vi "ABB configure system.vi"() -> ()   [LabVIEW 2017]
uses:
  ABB global.vi
panel:
  in  "Altitude (m)":dbl
  in  "Max Winding temp Rise (°C)":dbl
  in  "Simulate cDAQ":bool
  in  "Power Analyser":bool
  in  "Exit":bool
  in  "Change password":bool
  in  "Select data Folder":bool
  out "Data Folder":path
  in  "Simulate Norma":bool
  in  "GPIB Addresses":cluster{"Norma 5000":u8, "????":u8}={"Norma 5000"=1, "????"=1} {"????" min=1 max=31; "Norma 5000" min=1 max=31}
  # "Configure System"
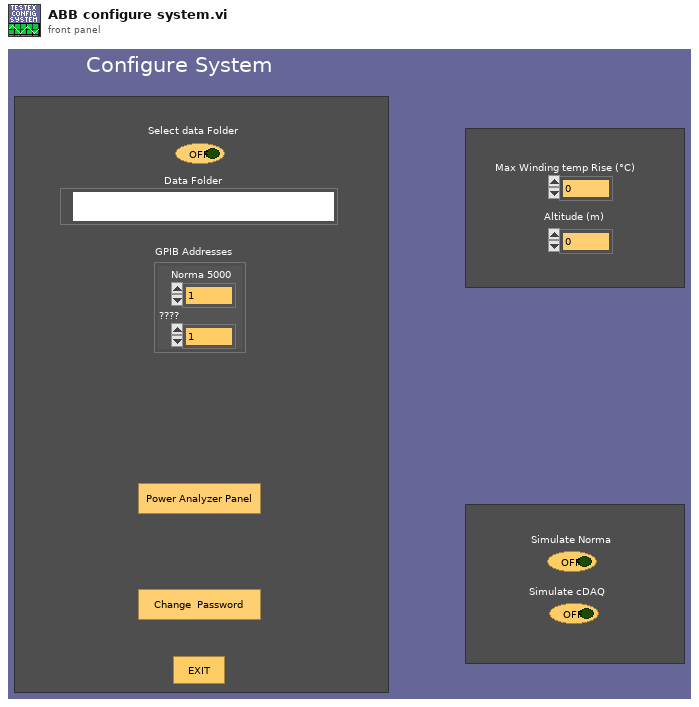
[diagram p1: front panel]
types:
  T1 = cluster{"Simulate Norma":bool, "Norma 5000 Address":u8, "WebDaq IP Address":string, "Simulate cDAQ":bool}
  T2 = enum32{"existing file", "new file", "new or existing file", "existing dir", "new dir", "new or existing dir", "existing file (use LLBs)", "new file (use LLBs)", "new or existing file (use LLBs)", "new or existing file or directory (use LLBs)"}
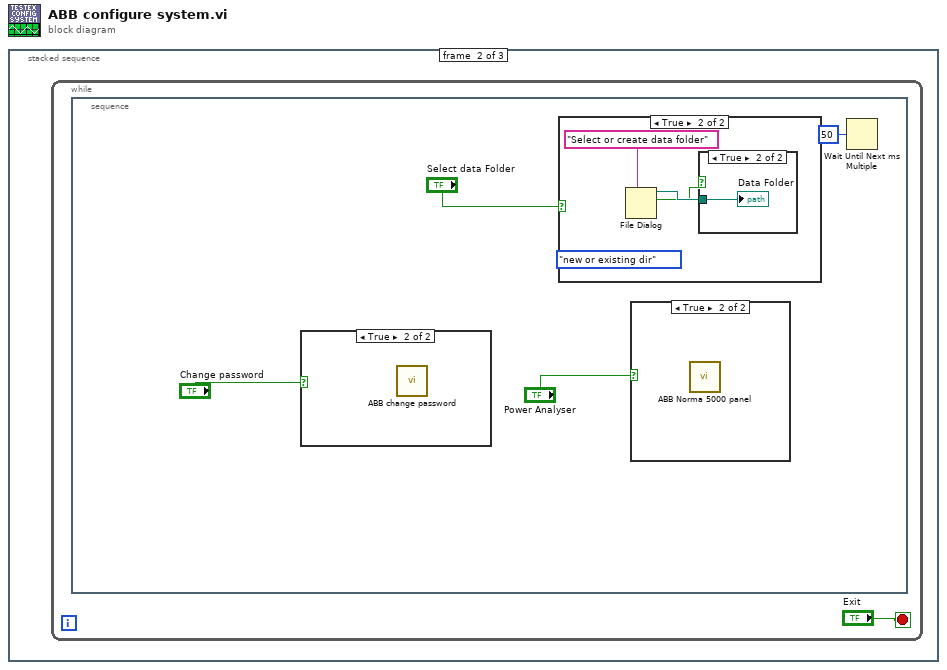
[diagram p0: block diagram]
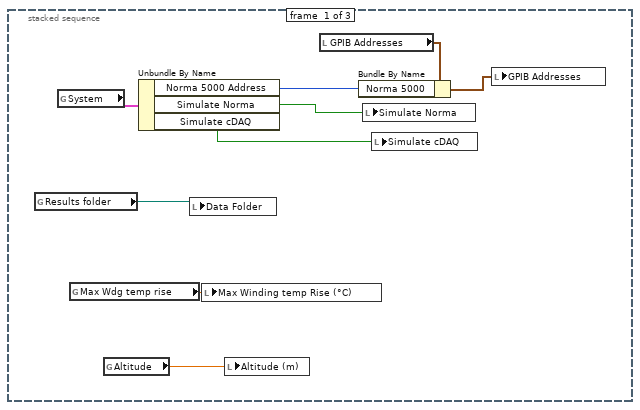
[diagram p2: hidden frame]
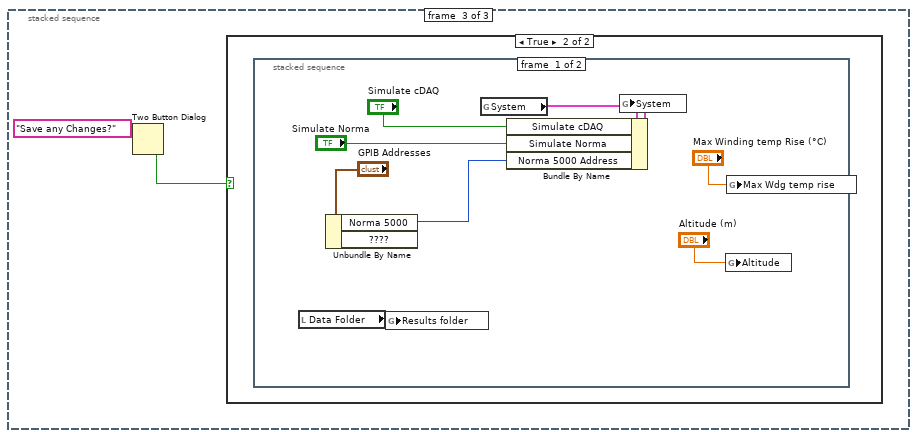
[diagram p7: hidden frame]
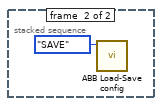
[diagram p9: hidden frame]
diagram:
  n1 = stacked-sequence {
    frame #0 {
      n2 = global read "ABB global.vi" "Results folder"() -> (w4:path)
      n3 = global read "ABB global.vi" "System"() -> (w9:T1)
      n4 = global read "ABB global.vi" "Max Wdg temp rise"() -> (w2:dbl)
      n5 = global read "ABB global.vi" "Altitude"() -> (w1:dbl)
      n6 = Unbundle By Name(w9) -> ("Norma 5000 Address"=w7:u8, "Simulate Norma"=w5:bool, "Simulate cDAQ"=w3:bool)
      n7 = local write "Data Folder"(w4) -> ()
      n8 = local write "Max Winding temp Rise (°C)"(w2) -> ()
      n9 = local write "Altitude (m)"(w1) -> ()
      n10 = local read "GPIB Addresses"() -> (w8:cluster{"Norma 5000":u8, "????":u8})
      n11 = Bundle By Name(cluster=w8, "Norma 5000"=w7) -> (w6:cluster{"Norma 5000":u8, "????":u8})
      n12 = local write "Simulate Norma"(w5) -> ()
      n13 = local write "Simulate cDAQ"(w3) -> ()
      n14 = local write "GPIB Addresses"(w6) -> ()
    }
    frame #1 {
      n15 = while {
        stop <- "Exit" stop-if-true
        n16 = stacked-sequence {
          frame #0 {
            n17 = case shown="True" "Change password" {
              frame False {
              }
              frame True {
                n18 = call "ABB change password.vi"() -> ()  [unwired: 5 in]
              }
            }
            n19 = case shown="True" "Select data Folder" {
              frame False {
              }
              frame True {
                (unwired) T2."new or existing dir" ("select mode (2)")
                n20 = File Dialog(7:"Select or create data folder" ("prompt")) -> (2:w15:bool, 3:w16:path)  [unwired: 6 in, 2 out]
                n21 = case shown="True" w15 {
                  tunnel: w16 -> [_ w18]
                  frame False {
                  }
                  frame True {
                    "Data Folder" <- w18
                  }
                }
              }
            }
            n22 = case shown="True" "Power Analyser" {
              frame False {
              }
              frame True {
                n23 = call "ABB Norma 5000 panel.vi"() -> ()  [unwired: 1 in]
              }
            }
            n24 = Wait Until Next ms Multiple(millisecond multiple=u32 50) -> ()  [unwired: 1 out]
          }
        }
      }
    }
    frame #2 {
      n25 = Two Button Dialog(message="Save any Changes?") -> (T button?=w19:bool)  [unwired: 2 in]
      n26 = case shown="True" w19 {
        frame False {
        }
        frame True {
          n27 = stacked-sequence {
            frame #0 {
              n28 = local read "Data Folder"() -> (w25:path)
              n29 = Unbundle By Name("GPIB Addresses") -> ("Norma 5000"=w27:u8)  [unwired: 1 out]
              n30 = global write "ABB global.vi" "Results folder"(w25) -> ()
              n31 = global read "ABB global.vi" "System"() -> (w29:T1)
              n32 = Bundle By Name(cluster=w29, "Simulate cDAQ"="Simulate cDAQ", "Simulate Norma"="Simulate Norma", "Norma 5000 Address"=w27) -> (w26:T1)
              n33 = global write "ABB global.vi" "System"(w26) -> ()
              n34 = global write "ABB global.vi" "Altitude"("Altitude (m)") -> ()
              n35 = global write "ABB global.vi" "Max Wdg temp rise"("Max Winding temp Rise (°C)") -> ()
            }
            frame #1 {
              n36 = call "ABB Load-Save config.vi"("Mode"=enum16{"LOAD", "SAVE"}."SAVE") -> ()  [unwired: 11 in]
            }
          }
        }
      }
    }
  }
